vi "VerifyChecksum.vi"(1 "HEX String to Verify CheckSum":string) -> (0 "Success?":bool)   [LabVIEW 2014]
panel:
  out "Expected_Length":u8
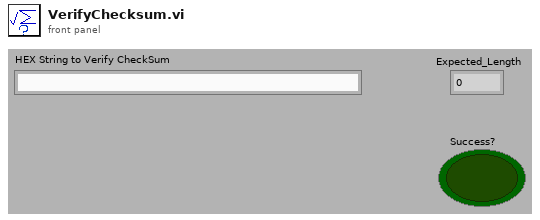
[diagram p1: front panel]
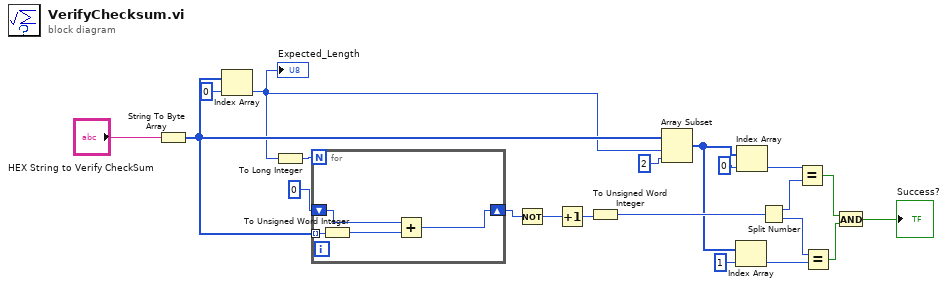
[diagram p0: block diagram]
diagram:
  n1 = String To Byte Array(string="HEX String to Verify CheckSum") -> (unsigned byte array=w13:u8[])
  n2 = Index Array(array=w13, index=0) -> (element=w12:u8)
  "Expected_Length" <- w12
  n3 = To Long Integer(number=w12) -> (32bit integer=w16:i32)
  n4 = for {
    N: w16 -> [_]
    tunnel: w13 -> [w25] mode=indexing
    shift-right: [w22] -> w14
    shift-left: u16 0 ("Numeric") -> [w23]
    n5 = To Unsigned Word Integer(number=w25) -> (unsigned 16bit integer=w24:u16)
    n6 = Add(x=w23, y=w24) -> (x+y=w22:u16)
  }
  n7 = Not(x=w14) -> (.not. x?=w21:u16)
  n8 = Increment(x=w21) -> (x+1=w20:u16)
  n9 = To Unsigned Word Integer(number=w20) -> (unsigned 16bit integer=w19:u16)
  n10 = Array Subset(array=w13, index=w12, length=2) -> (w8:u8[])
  n11 = Index Array(array=w8, index=1) -> (element=w5:u8)
  n12 = Index Array(array=w8, index=0) -> (element=w6:u8)
  n13 = Split Number(x=w19) -> (hi(x)=w10:u8, lo(x)=w4:u8)
  n14 = Equal?(x=w6, y=w10) -> (x = y?=w3:bool)
  n15 = Equal?(x=w4, y=w5) -> (x = y?=w2:bool)
  n16 = And(x=w3, y=w2) -> (x .and. y?=→"Success?":bool)
